vi "Generate_Array.vi"(1 "Dimensions":u32[](array[numeric])=[3, 5]) -> (0 "Array":bool[][](array[boolean]))   [LabVIEW 2015]
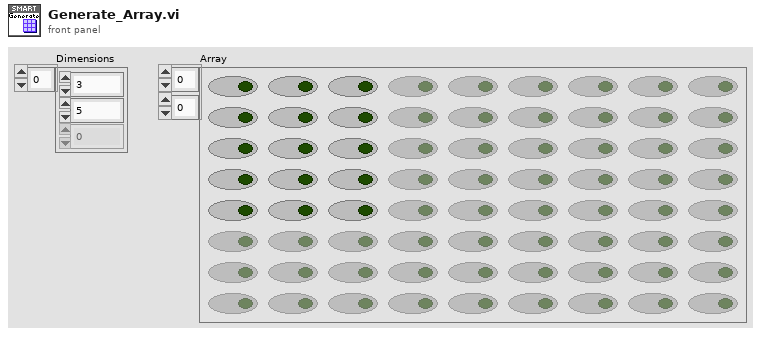
[diagram p1: front panel]
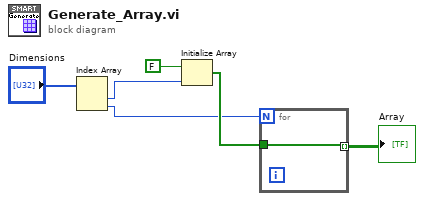
[diagram p0: block diagram]
diagram:
  n1 = Index Array(array="Dimensions") -> (element #1=w4:u32, element #2=w1:u32)  [unwired: 2 in]
  n2 = Initialize Array(FALSE, w4) -> (w3:bool[])
  n3 = for {
    N: w1 -> [_]
    tunnel: w3 -> [w7]
    tunnel: [w7] -> w2 mode=indexing
  }
  "Array" <- w2
